vi "Update display target.vi"(8 "error in (no error)":errorcluster, 11 "StageSPIM in":refnum<class "StageSPIM.lvclass">) -> (0 "error out":errorcluster, 3 "StageSPIM out":refnum<class "StageSPIM.lvclass">)   [LabVIEW 2012, in "StageSPIM.lvclass"]
uses:
  StageSPIM.lvclass
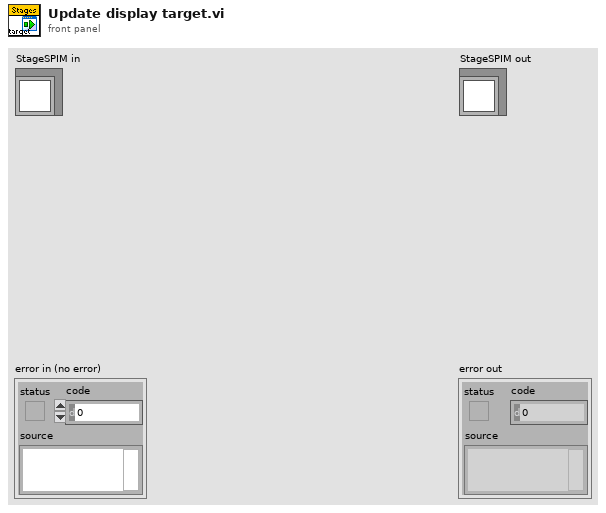
[diagram p1: front panel]
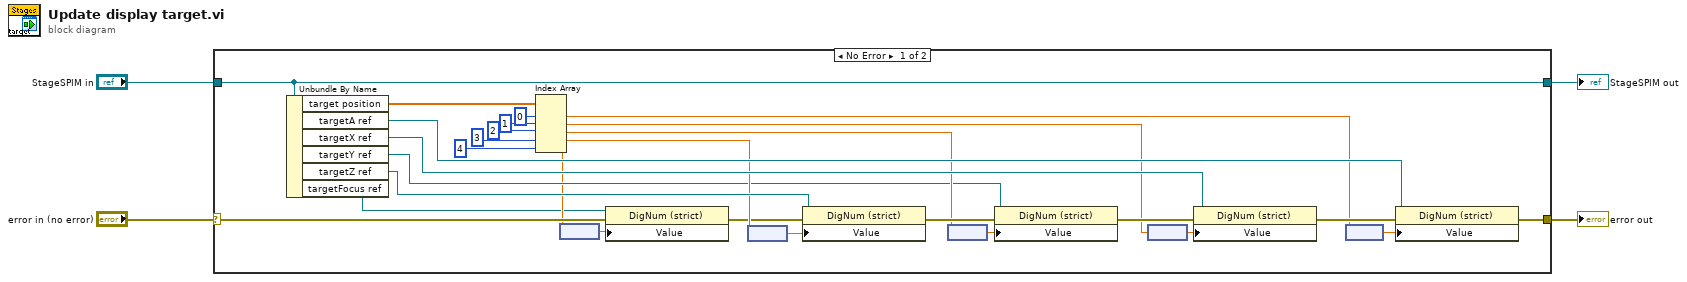
[diagram p0: block diagram]
diagram:
  n1 = case shown="No Error" "error in (no error)" {
    selector: "error in (no error)" -> [w9 w34]
    tunnel: [w12 w34] -> w3
    tunnel: [w13 w33] -> w1
    tunnel: "StageSPIM in" -> [w13 w33]
    frame No Error {
      n2 = Unbundle By Name(w13) -> ("target position"=w32:dbl[], "targetA ref"=w25:refnum<vi>, "targetX ref"=w26:refnum<vi>, "targetY ref"=w11:refnum<vi>, "targetZ ref"=w27:refnum<vi>, "targetFocus ref"=w5:refnum<vi>)
      n3 = Index Array(array=w32, index #1=0 ("index"), index #2=1 ("index"), index #3=2 ("index"), index #4=3 ("index"), index #5=4 ("index")) -> (element #1=w14:dbl, element #2=w16:dbl, element #3=w18:dbl, element #4=w20:dbl, element #5=w6:dbl)
      n4 = node(w6) -> (w7:dbl[unit])
      n5 = property class="DigNum (strict)"(reference=w5, error in=w9, "Value"=w7) -> (error out=w8:errorcluster)  [unwired: 1 out]
      n6 = node(w20) -> (w21:dbl[unit])
      n7 = property class="DigNum (strict)"(reference=w27, error in=w8, "Value"=w21) -> (error out=w24:errorcluster)  [unwired: 1 out]
      n8 = node(w18) -> (w19:dbl[unit])
      n9 = property class="DigNum (strict)"(reference=w11, error in=w24, "Value"=w19) -> (error out=w23:errorcluster)  [unwired: 1 out]
      n10 = node(w16) -> (w17:dbl[unit])
      n11 = property class="DigNum (strict)"(reference=w26, error in=w23, "Value"=w17) -> (error out=w22:errorcluster)  [unwired: 1 out]
      n12 = node(w14) -> (w15:dbl[unit])
      n13 = property class="DigNum (strict)"(reference=w25, error in=w22, "Value"=w15) -> (error out=w12:errorcluster)  [unwired: 1 out]
    }
    frame Error {
    }
  }
  "error out" <- w3
  "StageSPIM out" <- w1
